vi "hwOperation Test.vi"() -> ()   [LabVIEW 2016]
uses:
  Modules/DAQ-Config/Controls/PSCHN_Card Para.ctl
  Modules/DAQ-Config/Controls/PSCHN_Channel Para.ctl
  Modules/DAQ-Device/Hardware Drivers/QX/hw_QX_hwDriverRef.ctl
  C:/Users/CL/Desktop/ZcDAQprj0811/ZcDAQprj/Modules/DAQ-Device/Hardware Drivers/QX/HBM LabVIEW Driver/DLLs/Hbm.Api.Common.dll
  Modules/DAQ-Device/Hardware Drivers/QX/HBM LabVIEW Driver/DLLs/Hbm.Api.Common.dll
panel:
  out "hwDriverRef out":T1
  out "Frequency":dbl
  in  "Update Cfg":bool
  in  "Cancel Button":bool
  in  "read hwCfg":bool
  in  "Conn":bool
  in  "Devs Info":T2[](array[typedef])
  out "error out":errorcluster
  out "Connect?":bool
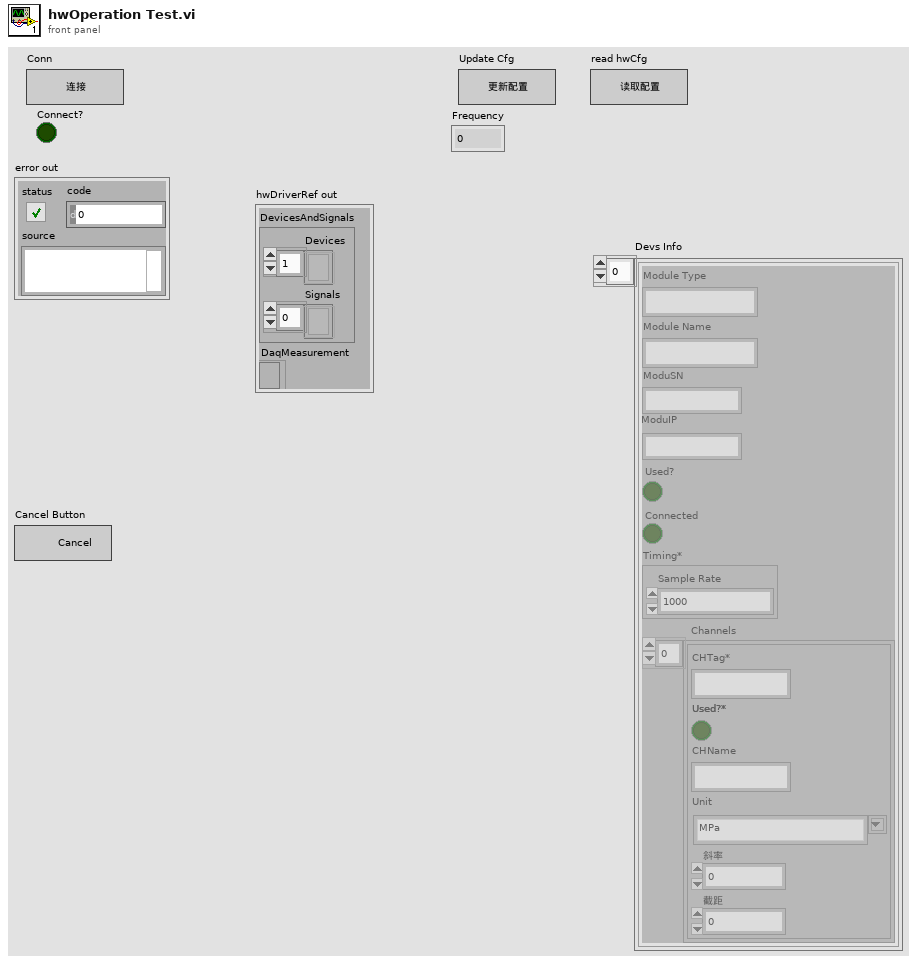
[diagram p1: front panel]
types:
  T1 = typedef "hw_QX_hwDriverRef.ctl" = cluster{"DevicesAndSignals":cluster{"Devices":refnum<k24>[], "Signals":refnum<k24>[]}, "DaqMeasurement":refnum<k24>}
  T2 = typedef "PSCHN_Card Para.ctl" = cluster{"Module Type":string, "Module Name":string, "ModuSN":string, "ModuIP":string, "Used?":bool, "Connected":bool, "Timing*":cluster{"Sample Rate":dbl}, "Channels":T3[]}
  T3 = typedef "PSCHN_Channel Para.ctl" = cluster{"CHTag*":string, "Used?*":bool, "CHName":string, "Unit":string, "斜率":dbl, "截距":dbl}
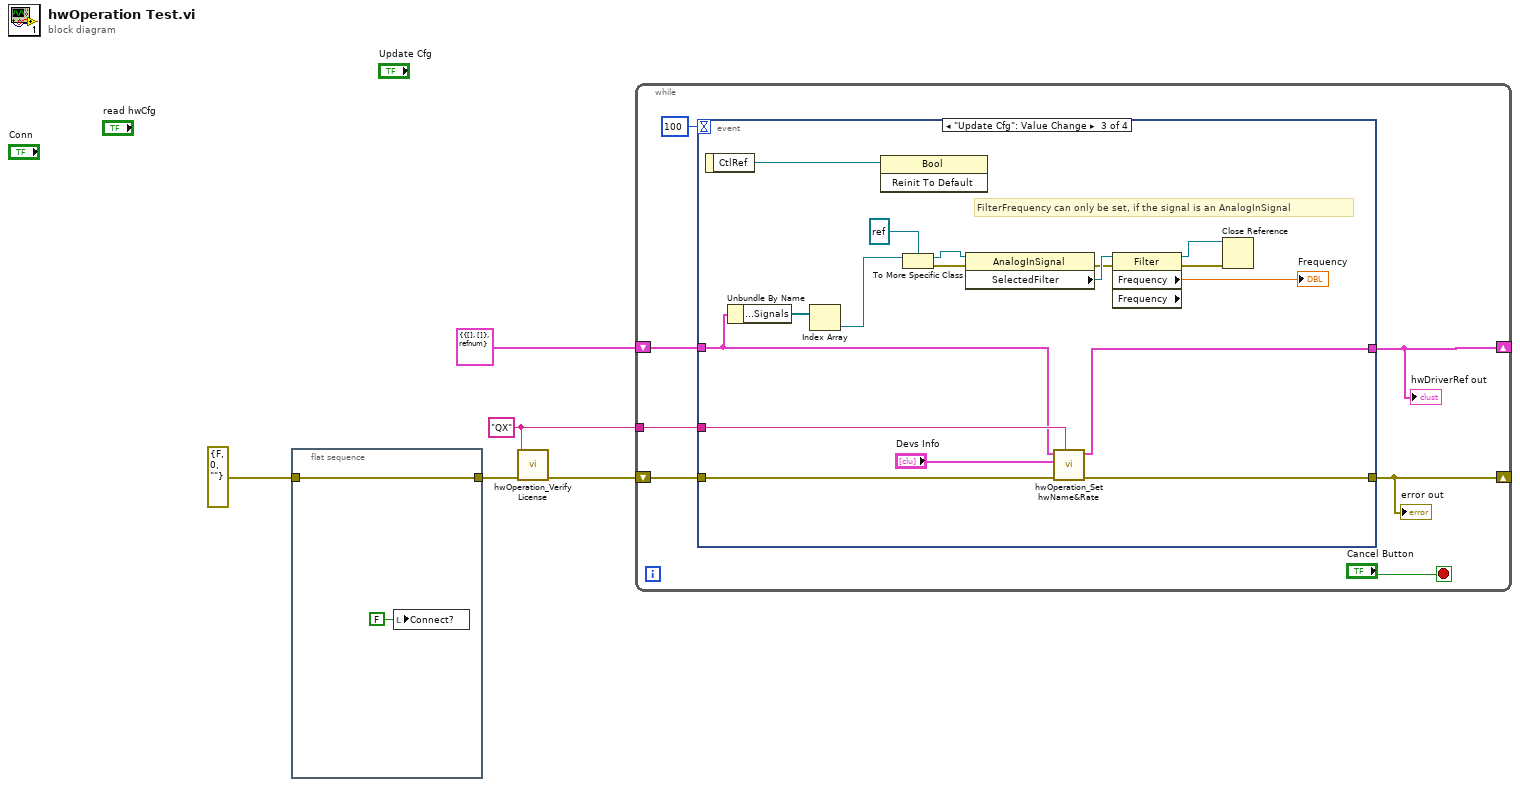
[diagram p0: block diagram]
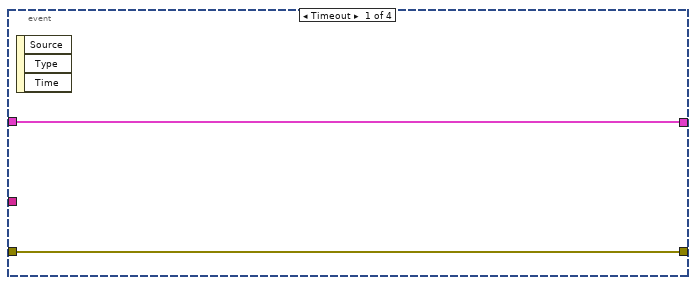
[diagram p2: hidden frame]
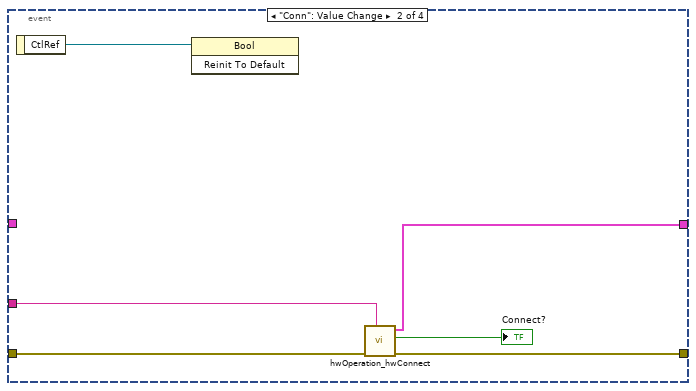
[diagram p3: hidden frame]
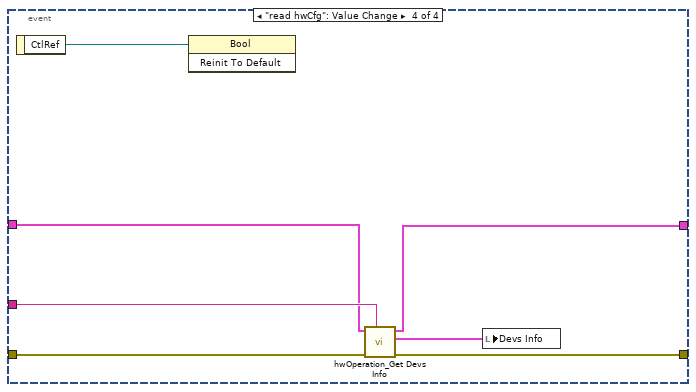
[diagram p4: hidden frame]
diagram:
  w4 = "QX" ("hwType")
  n1 = flat-sequence {
    tunnel: [w7] -> w3
    tunnel: errorcluster {"status"=FALSE, "code"=0, "source"=""} ("Error in") -> [w7]
    frame #0 {
      n2 = local write "Connect?"(FALSE ("Connect?")) -> ()
    }
  }
  n3 = call "hwOperation_Verify License.vi"("hwType"=w4, "Error in"=w3) -> ("Error out"=w5:errorcluster)  [unwired: 8 in]
  n4 = while {
    tunnel: w4 -> [w12]
    shift-right: [w11] -> _
    shift-left: w5 -> [w13]
    shift-right: [w8] -> _
    shift-left: T1 {"DevicesAndSignals"={"Devices"=[], "Signals"=[]}, "DaqMeasurement"=refnum} ("hwDriverRef out") -> [w9]
    stop <- "Cancel Button" stop-if-true
    n5 = event shown="[2] \"Update Cfg\": Value Change" {
      selector: _ -> [_ _ _ _]
      dyn-events: _ -> [_ _ _ _]
      timeout: 100 -> [_ _ _ _]
      tunnel: w13 -> [w16 w21 w37 w45]
      tunnel: w12 -> [_ w19 w36 w44]
      tunnel: [w16 w18 w38 w43] -> w11
      tunnel: [w15 w17 w35 w42] -> w8
      tunnel: w9 -> [w15 _ w30 w40]
      event Timeout {
        n6 = event-data() -> ()  [unwired: 1 in, 3 out]
      }
      event "Conn": Value Change {
        n7 = event-data() -> ("CtlRef"=w22:refnum<vi>)  [unwired: 1 in]
        n8 = invoke class="Bool" method="Reinit To Default"(reference=w22) -> ()  [unwired: 2 in, 3 out]
        n9 = call "hwOperation_hwConnect.vi"("hwType"=w19, "error in (no error)"=w21) -> ("error out"=w18:errorcluster, "Connect?"=→"Connect?":bool, "hwDriverRef"=w17:T1)  [unwired: 7 in]
      }
      event "Update Cfg": Value Change {
        # "FilterFrequency can only be set, if the signal is an AnalogInSignal"
        n10 = event-data() -> ("CtlRef"=w39:refnum<vi>)  [unwired: 1 in]
        n11 = Unbundle By Name(w30) -> ("DevicesAndSignals.Signals"=w29:refnum<k24>[])
        n12 = Index Array(array=w29) -> (element=w28:refnum<k24>)  [unwired: 1 in]
        n13 = invoke class="Bool" method="Reinit To Default"(reference=w39) -> ()  [unwired: 2 in, 3 out]
        n14 = To More Specific Class(target class=refnum<k24> refnum (".NET (Referenz)"), reference=w28) -> (specific class reference=w32:refnum<k24>, error out=w31:errorcluster)  [unwired: 1 in]
        n15 = property on="Eigenschaftsknoten" class="AnalogInSignal"(reference=w32, error in=w31) -> (error out=w26:errorcluster, "SelectedFilter"=w27:refnum<k24>)  [unwired: 1 out]
        n16 = call "hwOperation_Set hwName&Rate.vi"("hwType"=w36, "error in"=w37, "Devs Info in"="Devs Info", "hwDriverRef in"=w30) -> ("error out"=w38:errorcluster, "hwDriverRef out"=w35:T1)  [unwired: 5 in, 1 out]
        n17 = property on="Eigenschaftsknoten" class="Filter" props=["Frequency", "Frequency"](reference=w27, error in=w26) -> (reference out=w24:refnum<k24>, error out=w25:errorcluster, "Frequency"=→"Frequency":dbl)  [unwired: 1 out]
        n18 = Close Reference(reference=w24, error in (no error)=w25) -> ()  [unwired: 1 out]
      }
      event "read hwCfg": Value Change {
        n19 = event-data() -> ("CtlRef"=w46:refnum<vi>)  [unwired: 1 in]
        n20 = invoke class="Bool" method="Reinit To Default"(reference=w46) -> ()  [unwired: 2 in, 3 out]
        n21 = call "hwOperation_Get Devs Info.vi"("hwType"=w44, "error in"=w45, "hwDriverRef in"=w40) -> ("error out"=w43:errorcluster, "Devs Info"=w41:T2[], "hwDriverRef out"=w42:T1)  [unwired: 6 in]
        n22 = local write "Devs Info"(w41) -> ()
      }
    }
    "error out" <- w11
    "hwDriverRef out" <- w8
  }
